vi "Execute_Single_Process.vi"(0 "Tab Control":T5, 1 "MaskParam 2":refnum<vi>, 5 "Parameter":variant, 7 "ImageIn":T3, 9 "ExtractImageControl":T3, 11 "error in (no error)":errorcluster, 12 "OperatorImage":T3) -> (3 "MaskParam 4":refnum<vi>, 4 "ProcessSettingOut":T6={"Enum_PreProcess"=enum."CamAttributes", "Parameter"=""}, 6 "ExtractImage":T3, 10 "Image Out":T3(plugin-control), 14 "OperatorImageOut":T3, 15 "error out":errorcluster)   [LabVIEW 2019]
uses:
  <vilib>/vision/NI_Vision_Development_Module.lvlib
  Controls/Process_Setting.ctl
  Controls/OperatorsParam_Type.ctl
  Controls/GrayMorphologyParam_Type.ctl
  Controls/LookupTableParam.ctl
  Controls/ParticleFilterParam_Type.ctl
  Controls/MaskParam_Type.ctl
  Ctrl/VisionProcessName.ctl
  <vilib>/vision/Image Controls.llb/IMAQ Image.ctl
  Controls/UI_Process_Type.ctl
  Controls/FiltersParam_Type.ctl
  Controls/BinaryMonoParam_Type.ctl
  Controls/ExtractPlanParam_Type.ctl
panel:
  in  "ExtractPlanParam":T1={"Color Plane"=enum."Green"}
  in  "BinaryMonoParam 2":T2={"Look For"=enum."Bright Objects", "Threshold"={136.0, 255.0}} {"Threshold" scale=0.0..255.0}
  in  "FiltersParam":T4={"Kernel"=[[1.0, 1.0, 1.0], [1.0, 1.0, 1.0], [1.0, 1.0, 1.0]], "Kernel Size"=0, "Filter Size X"=0, "Filter Size Y"=0, "Tolerance %"=0, "Divider"=0.0, "FilterFunction"=enum."Smoothing - Low Pass", "Sigma"=0.0, "LThres"=0.0, "HThresh"=0.0, "Windows Size"=0} {"Kernel Size" min=3 max=7 step=2}
  # "Minimum"
  # "Maximum"
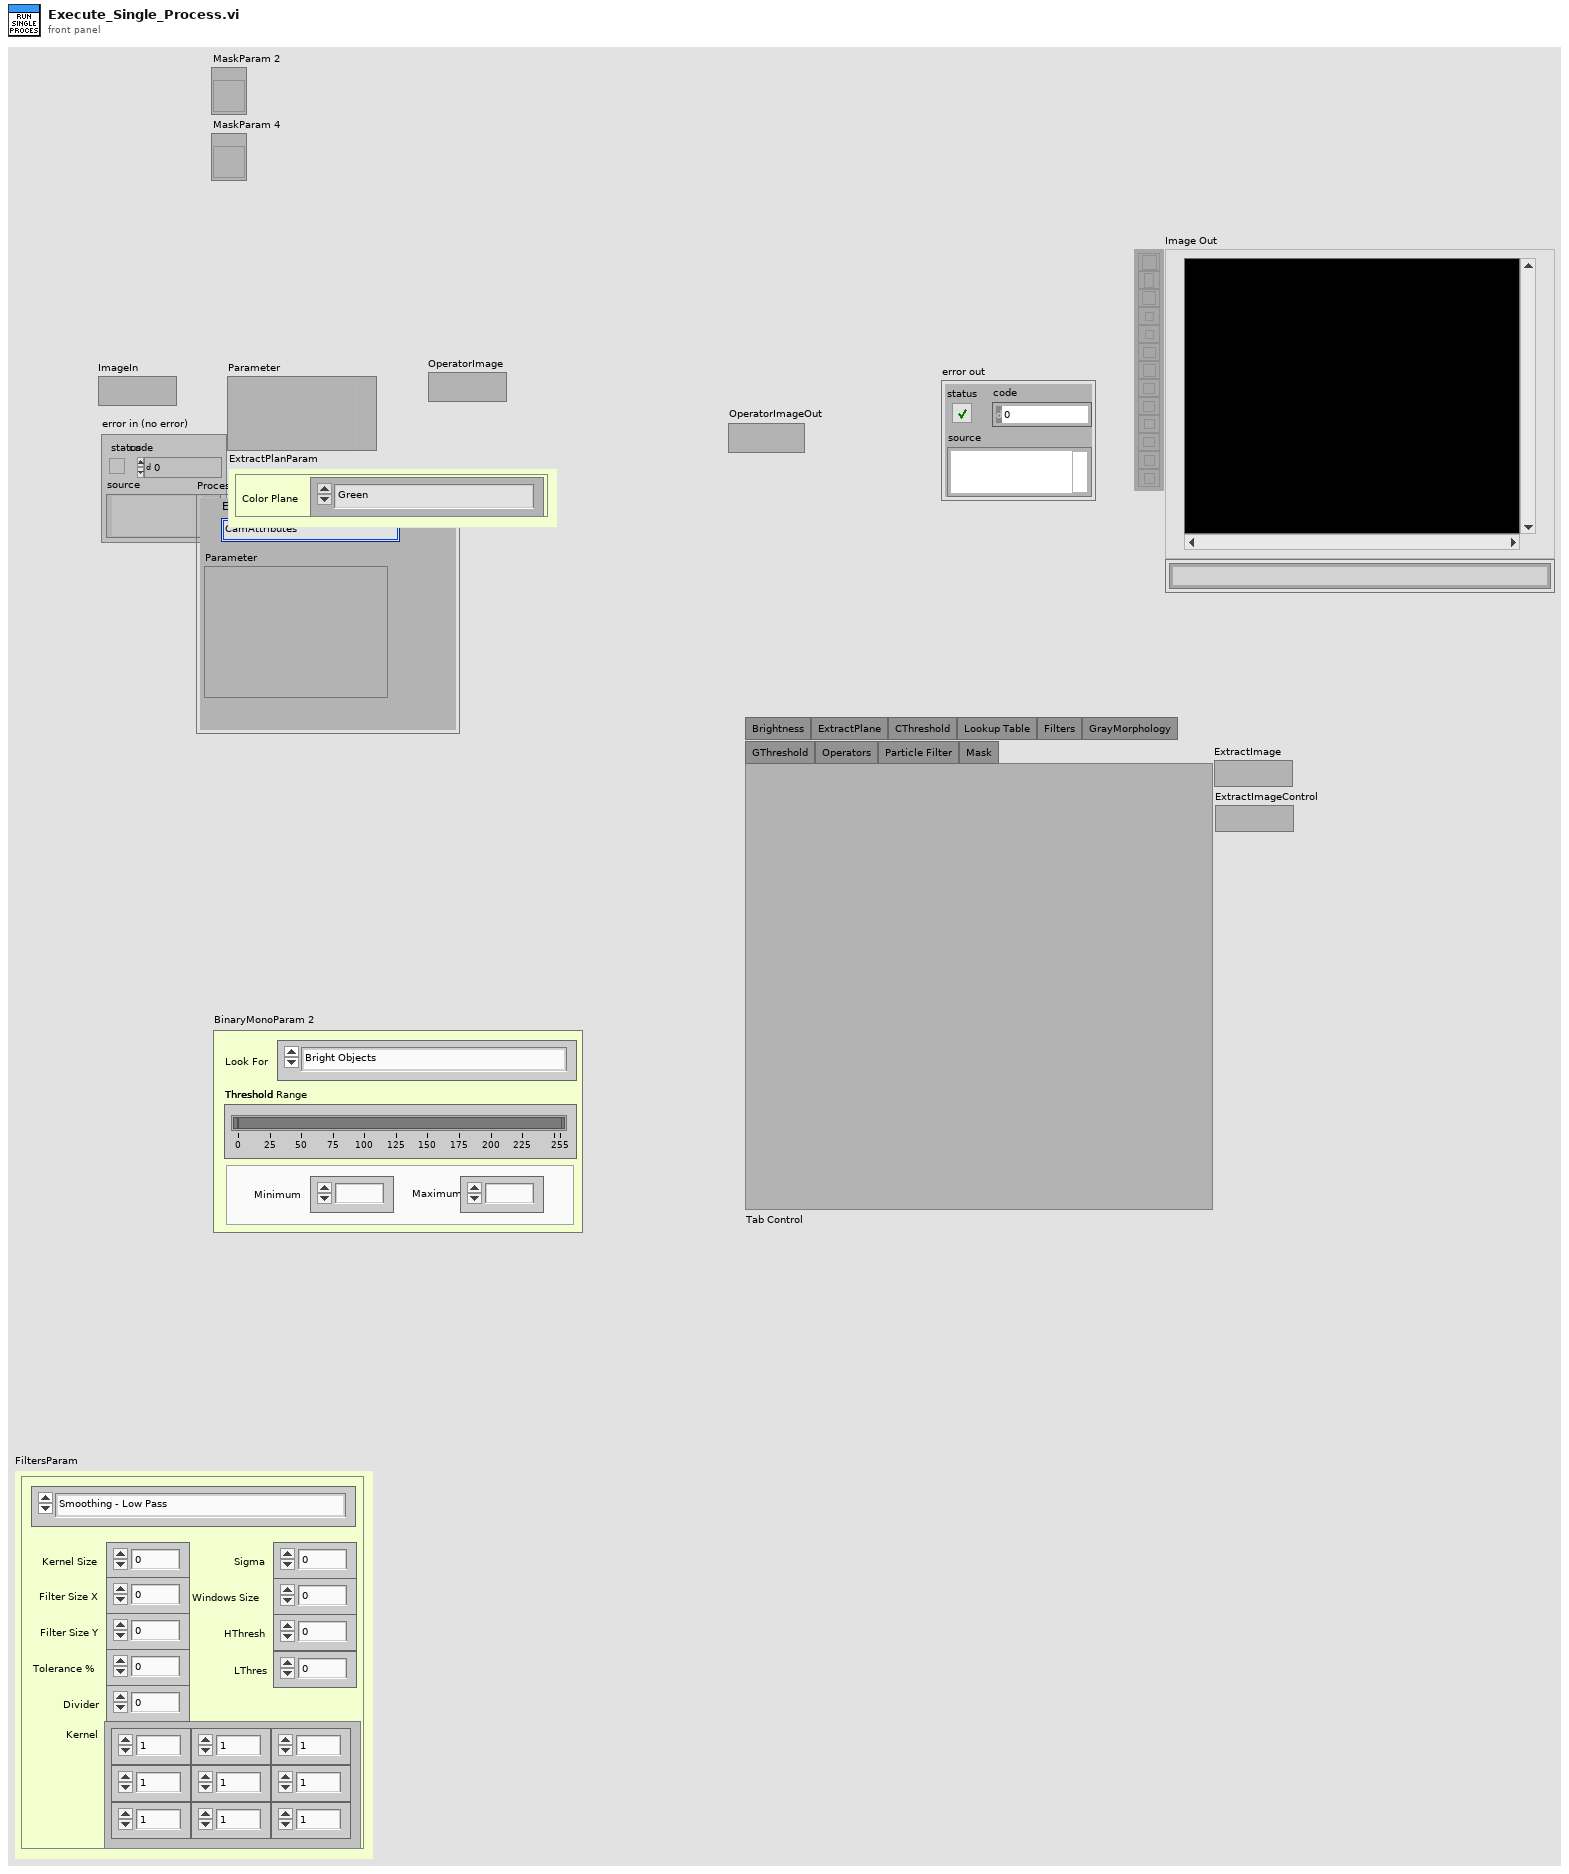
[diagram p1: front panel]
types:
  T1 = typedef "ExtractPlanParam_Type.ctl" = cluster{"Color Plane":enum16{"Red", "Green", "Blue", "Hue", "Saturation", "Luminance", "Value", "Intensity"}}
  T2 = typedef "BinaryMonoParam_Type.ctl" = cluster{"Look For":enum16{"Bright Objects", "Dark Objects", "Gray Objects"}, "Threshold":cluster{dbl, dbl}}
  T3 = typedef "IMAQ Image.ctl" = refnum<image>
  T4 = typedef "FiltersParam_Type.ctl" = cluster{"Kernel":sgl[][], "Kernel Size":i32, "Filter Size X":i32, "Filter Size Y":i32, "Tolerance %":i32, "Divider":sgl, "FilterFunction":enum16{"Smoothing - Low Pass", "Smoothing - Local Average", "Smoothing - Guassian", "Smoothing - Median", "------------------------------------", "Edge Detection - Laplacian", "Edge Detection - Diff", "Edge Detection - Prewitt", "Edge Detection - Sobel", "Edge Detection - Roberts", "Edge Detection - Canny", "Edge Detection - Gradient", "Edge Detection - Sigma", "----------------------------------------", "Convolution - Highlight Details", "Convolution - Custom"}, "Sigma":sgl, "LThres":sgl, "HThresh":sgl, "Windows Size":i32}
  T5 = typedef "UI_Process_Type.ctl" = enum32{"None", "Brightness", "ExtractPlane", "CThreshold", "Lookup Table", "Filters", "GrayMorphology", "GThreshold", "Operators", "Particle Filter", "Mask"}
  T6 = typedef "Process_Setting.ctl" = cluster{"Enum_PreProcess":T7, "Parameter":string}
  T7 = typedef "VisionProcessName.ctl" = enum16{"*CamParameter*", "CamAttributes", "*Preprocess*", "CG_Brightness", "C_Plane Extraction", "C_Threshold", "G_Lookup Table", "G_Threshold"}
  T8 = typedef "OperatorsParam_Type.ctl" = cluster{"Actions":enum16{"Add", "Subtract", "Multiply", "Divide", "Multiply Divide", "Modulo", "Absolutio Difference", "---------------------------------", "And", "Not And", "Or", "Not Or", "Exclusive Or", "Not Exclusive Or", "Logical Difference", "----------------------------------", "Mask"}, "Select Mode:":enum32{"Constant", "Image"}, "Color Box":u32, "Image Path":path}
  T9 = typedef "GrayMorphologyParam_Type.ctl" = cluster{"Operation":enum32{"AutoM", "Close", "Dilate", "Erode", "Gradient", "Gradient in", "Gradient out", "HitMiss", "Open", "PClose", "POpen", "Thick", "Thin"}, "Structuring Element":i32[][], "Square/Hexa (Square)":bool, "Number of iterations":i32}
  T10 = enum32{"Differentiation", "Gradient", "Prewitt", "Roberts", "Sigma", "Sobel"}
  T11 = typedef "LookupTableParam.ctl" = cluster{"Function":enum16{"Equalizer", "Reverse", "Logarithmic", "Exponential", "Square", "Square Root", "Power X", "Power 1/X"}, "Power Value":sgl}
  T12 = enum32{"Linear", "Log", "Exp", "Square", "Square root", "Power X", "Power 1/X"}
  T13 = typedef "ParticleFilterParam_Type.ctl" = cluster{"Selection Values":cluster{"Measurement Parameter":T14, "Range Lower Value":dbl, "Range Upper Value":dbl, "Range":bool, "Measurement Type":bool}[], "Keep/Remove Particles (F)":bool, "Reject Border? (F)":bool, "Fill Holes? (F)":bool, "Connectivity 4/8 (8)":bool}
  T14 = typedef "Particle Parameters" = i32
  T15 = enum16{"Red", "Green", "Blue", "Hue", "Saturation", "Luminance", "Value", "Intensity"}
  T16 = enum16{"Add", "Subtract", "Multiply", "Divide", "Multiply Divide", "Modulo", "Absolutio Difference", "---------------------------------", "And", "Not And", "Or", "Not Or", "Exclusive Or", "Not Exclusive Or", "Logical Difference", "----------------------------------", "Mask"}
  T17 = enum32{"AutoM", "Close", "Dilate", "Erode", "Gradient", "Gradient in", "Gradient out", "HitMiss", "Open", "PClose", "POpen", "Thick", "Thin"}
  T18 = enum16{"Smoothing - Low Pass", "Smoothing - Local Average", "Smoothing - Guassian", "Smoothing - Median", "------------------------------------", "Edge Detection - Laplacian", "Edge Detection - Diff", "Edge Detection - Prewitt", "Edge Detection - Sobel", "Edge Detection - Roberts", "Edge Detection - Canny", "Edge Detection - Gradient", "Edge Detection - Sigma", "----------------------------------------", "Convolution - Highlight Details", "Convolution - Custom"}
  T19 = cluster{"Filter Size X":i32, "Filter Size Y":i32, "Tolerance %":i32}
  T20 = cluster{"Filter Size X":i32, "Filter Size Y":i32, dbl}
  T21 = cluster{"Sigma":sgl, "HThresh":sgl, "LThres":sgl, "WindowSize":i32}
  T22 = enum16{"Equalizer", "Reverse", "Logarithmic", "Exponential", "Square", "Square Root", "Power X", "Power 1/X"}
  T23 = cluster{"histogram":u32[], "Minimal Value":sgl, "Maximal Value":sgl, "Starting Value":sgl, "Interval Width":sgl, "Mean Value":sgl, "Standard  Variation":sgl, "Area (pixels)":i32}
  T24 = typedef "Image Type" = u32
  T25 = cluster{"Measurement Parameter":T14, "Range Lower Value":dbl, "Range Upper Value":dbl, "Range":bool, "Measurement Type":bool}[]
  T26 = typedef "MaskParam_Type.ctl" = cluster{"Function":enum16{"Inside", "Outside"}, "ROI List":i32, "ROI":cluster{"Global Rectangle":i32[], "Contours":cluster{"Contour Type":u32, "ROI Type":u32, "Points":i32[]}[]}[], "Creat ROI":bool, "Delete ROI":bool, "Enabled/Disabled":bool, "Color Box":u32, "Last Mouse Position":cluster{"X":i32, "Y":i32}}
  T27 = cluster{"Global Rectangle":i32[], "Contours":cluster{"Contour Type":u32, "ROI Type":u32, "Points":i32[]}[]}[]
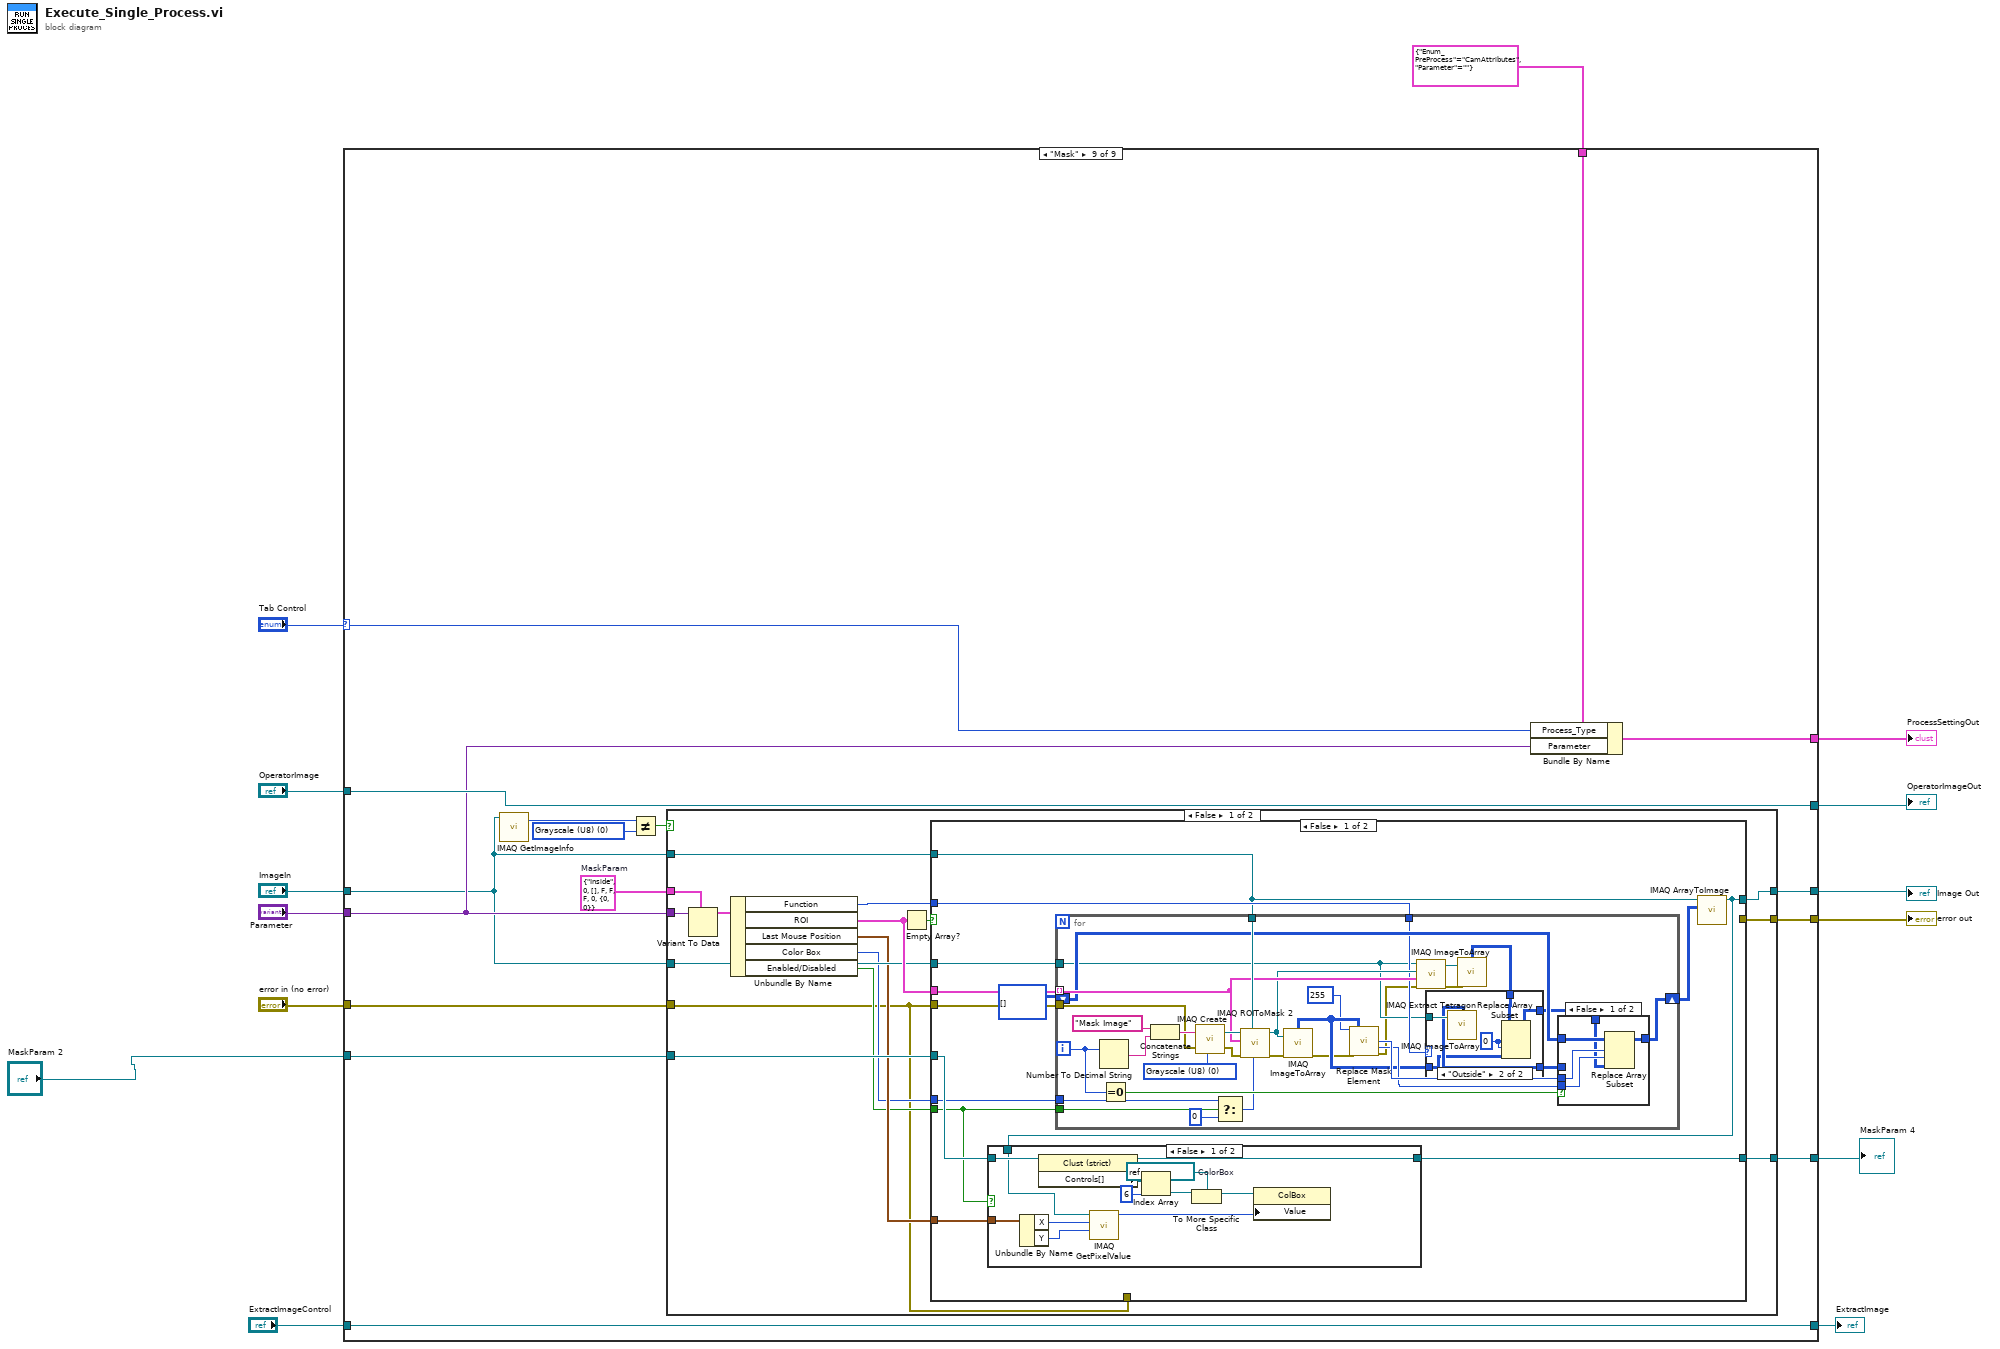
[diagram p0: block diagram]
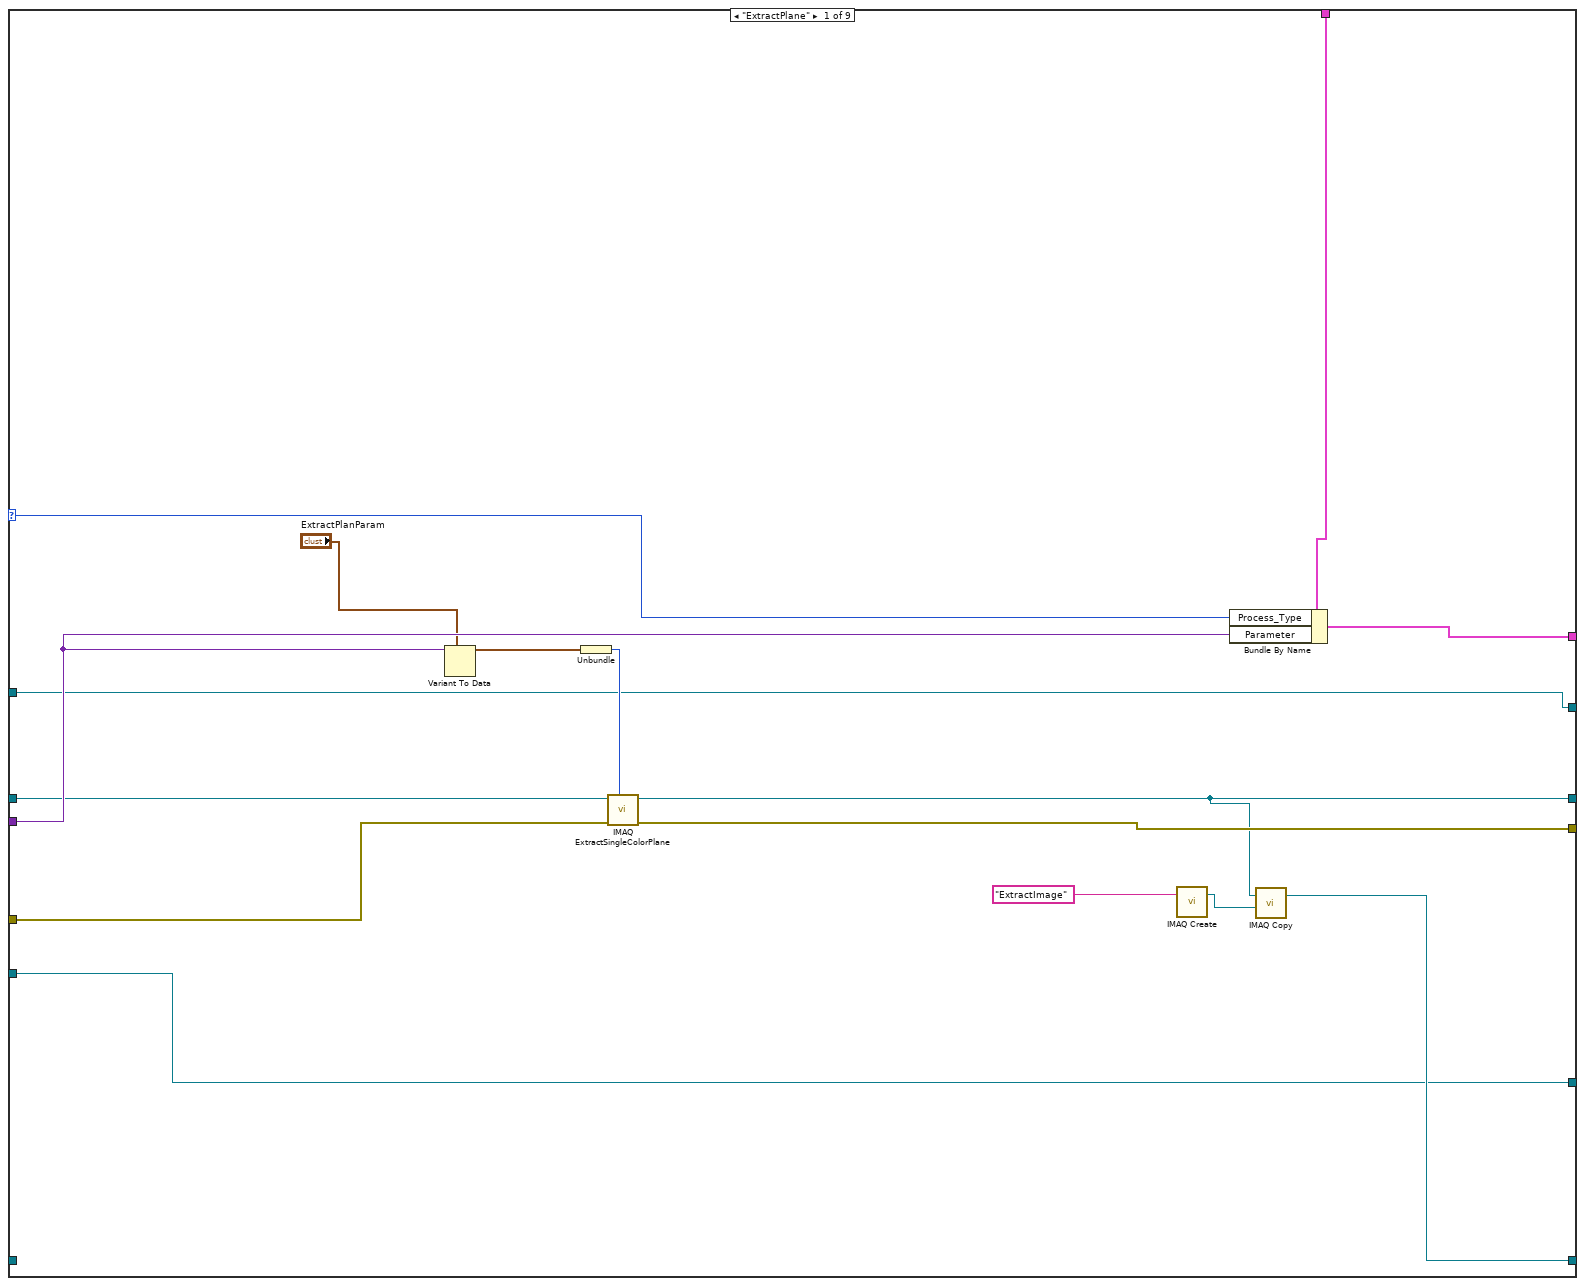
[diagram p2: hidden frame]
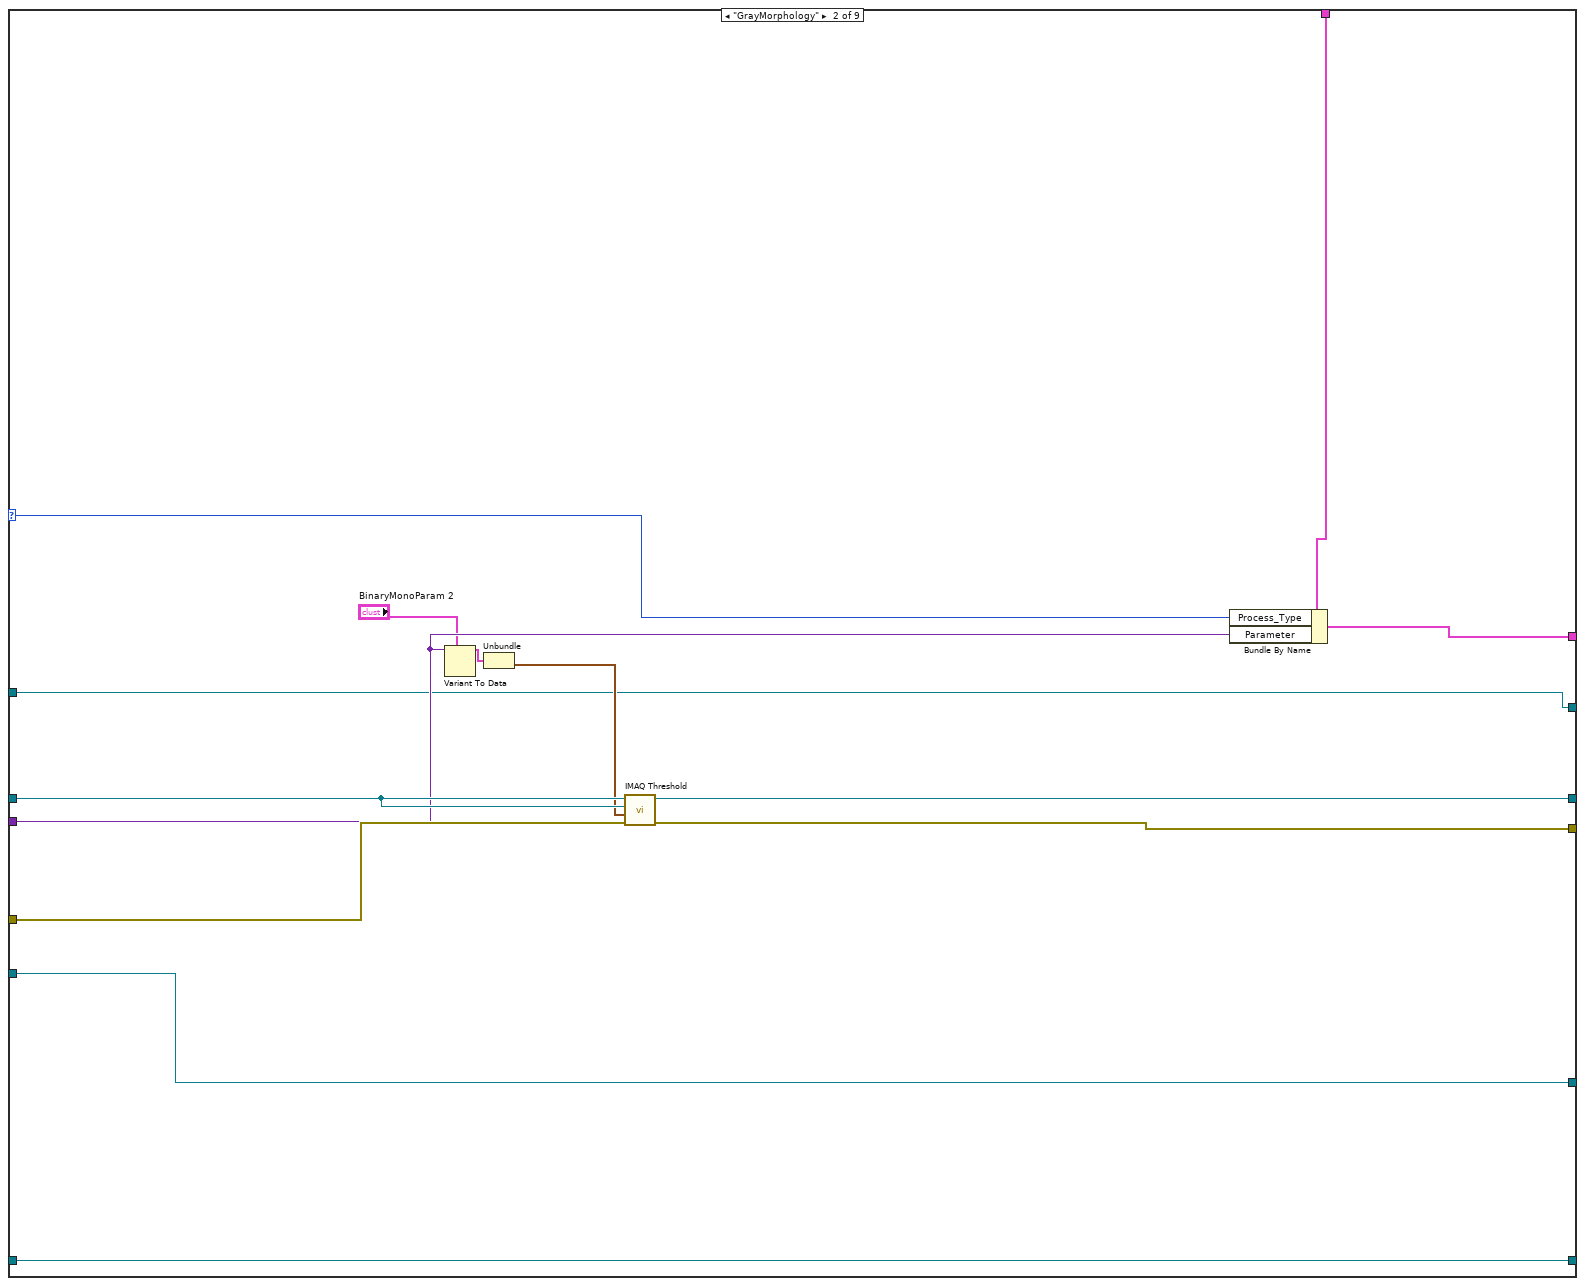
[diagram p3: hidden frame]
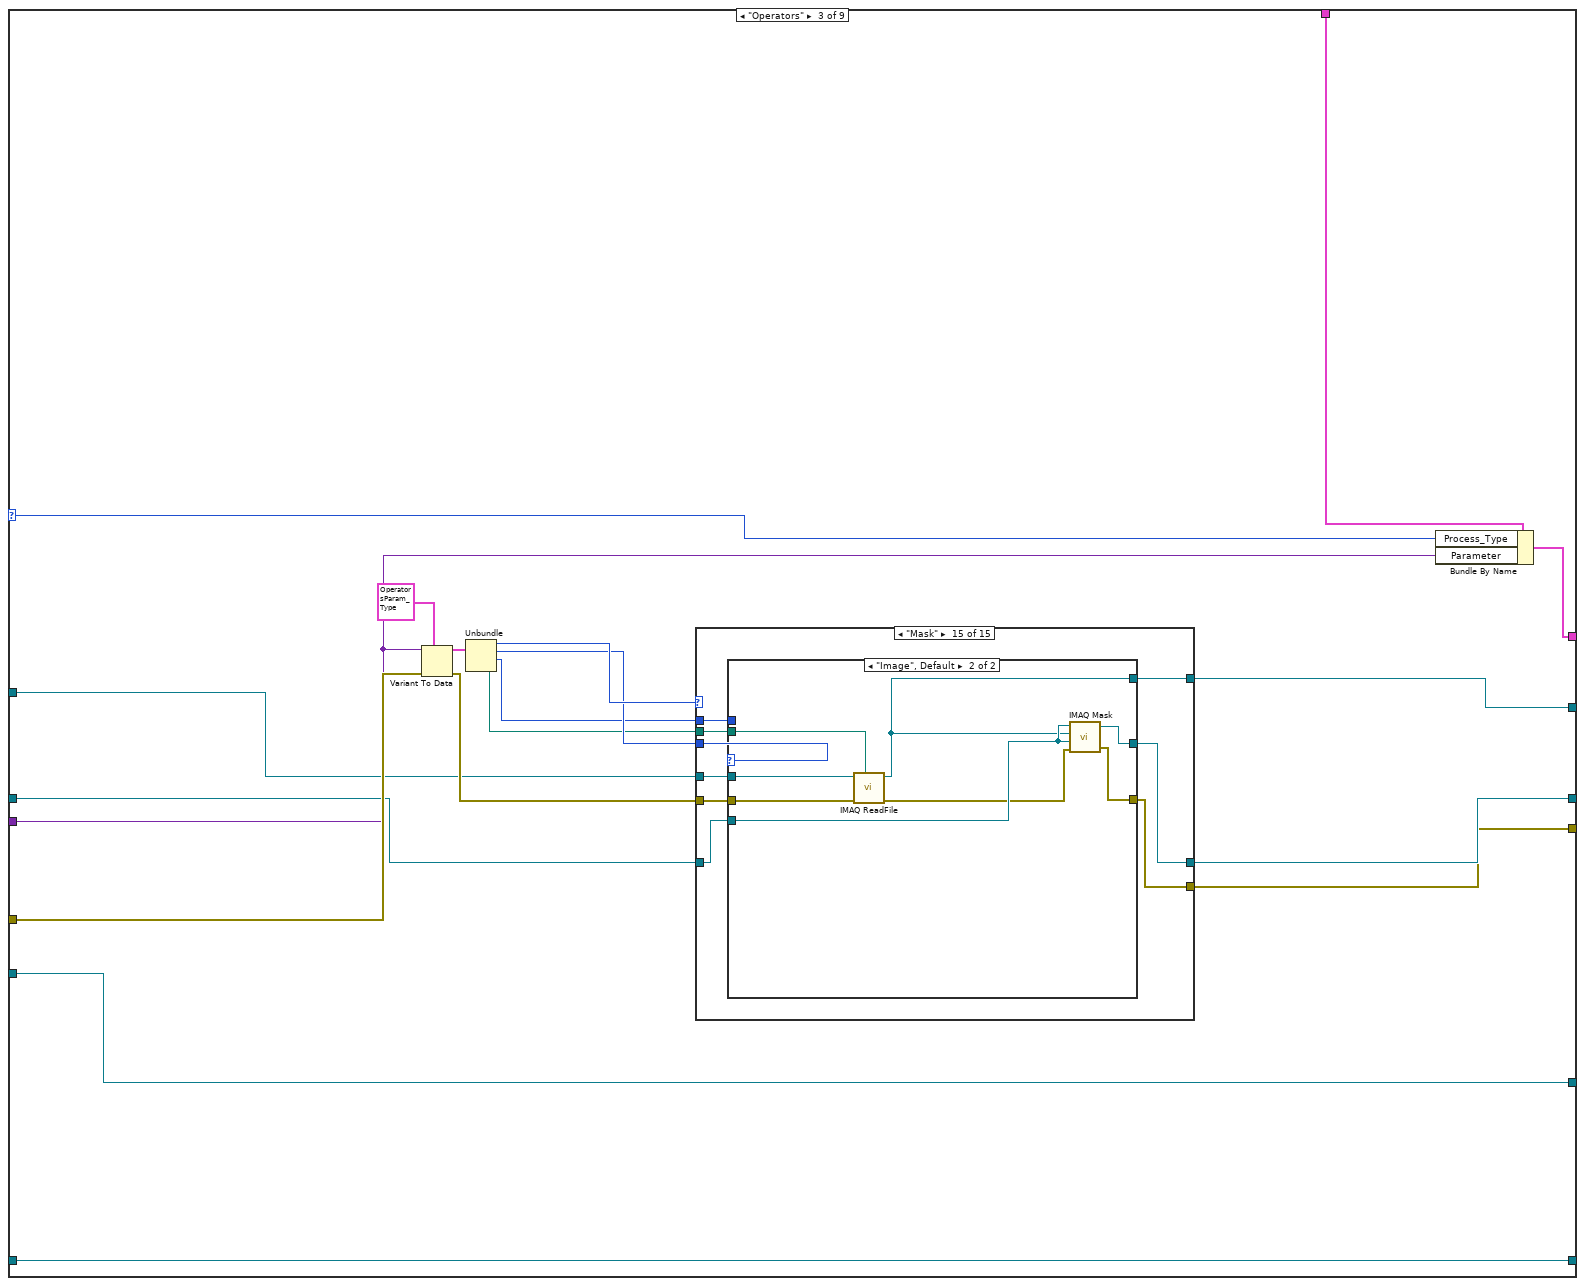
[diagram p4: hidden frame]
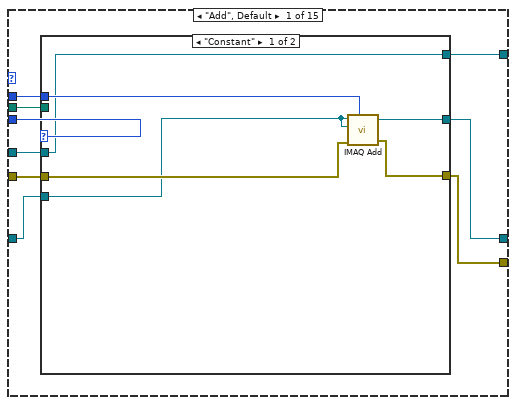
[diagram p5: hidden frame]
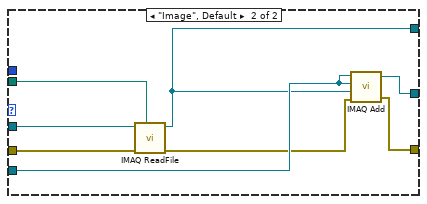
[diagram p6: hidden frame]
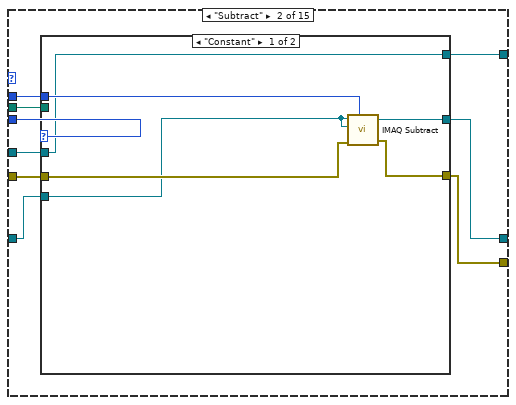
[diagram p7: hidden frame]
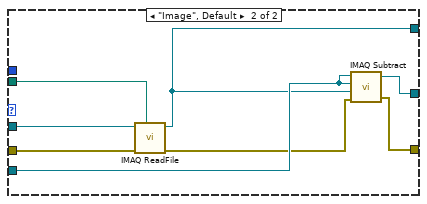
[diagram p8: hidden frame]
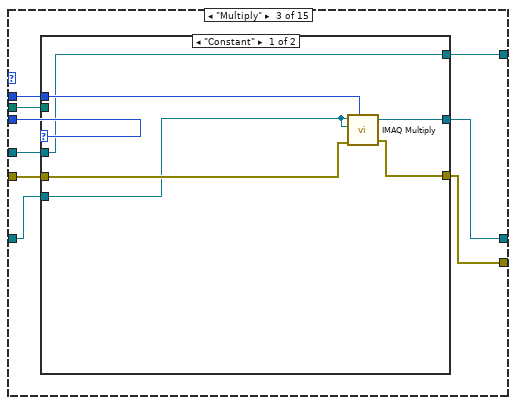
[diagram p9: hidden frame]
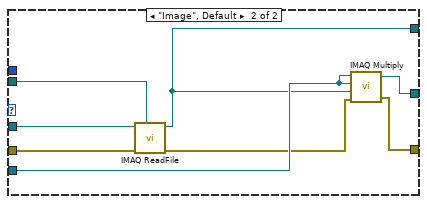
[diagram p10: hidden frame]
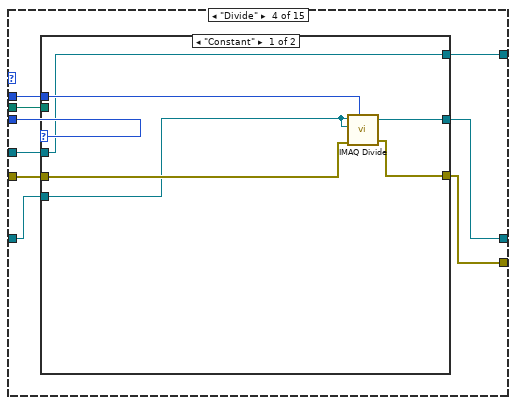
[diagram p11: hidden frame]
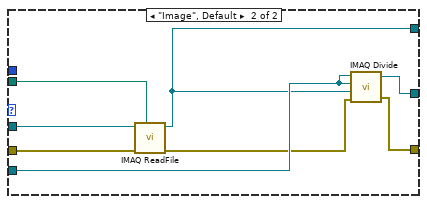
[diagram p12: hidden frame]
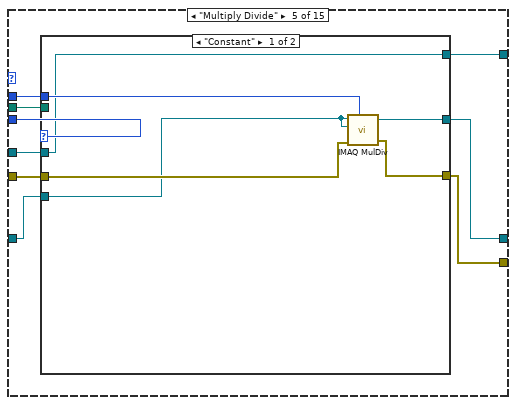
[diagram p13: hidden frame]
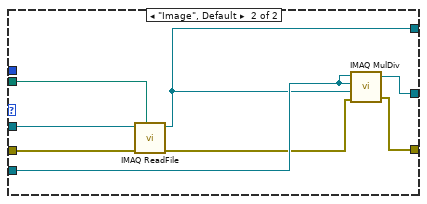
[diagram p14: hidden frame]
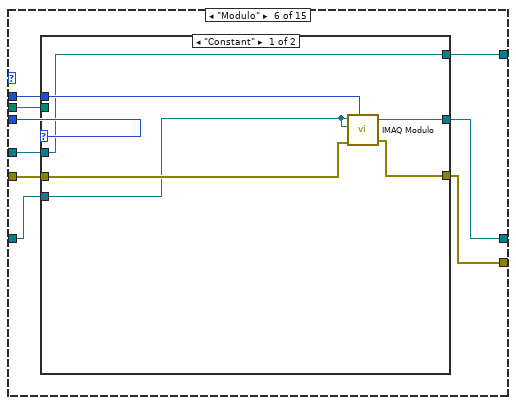
[diagram p15: hidden frame]
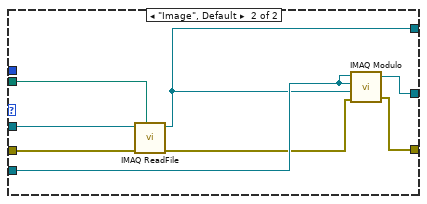
[diagram p16: hidden frame]
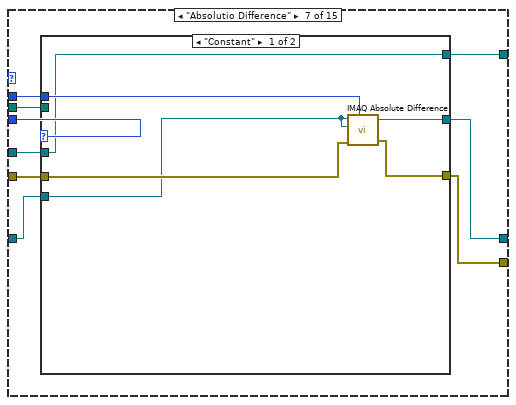
[diagram p17: hidden frame]
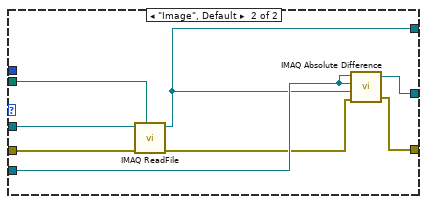
[diagram p18: hidden frame]
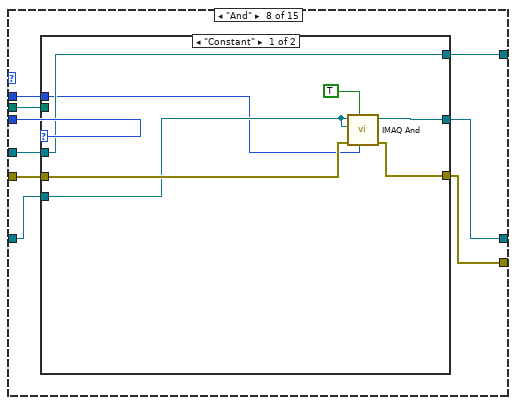
[diagram p19: hidden frame]
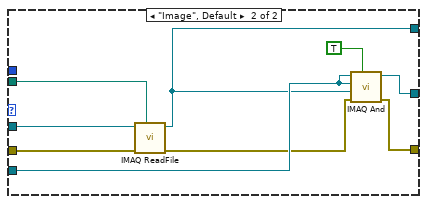
[diagram p20: hidden frame]
diagram:
  n1 = case shown="\"Mask\"" "Tab Control" {
    selector: "Tab Control" -> [w26 w42 w51 w423 w456 w584 w661 _ w680]
    tunnel: "ImageIn" -> [w22 w39 w60 w426 w448 w592 w657 w672 w673]
    tunnel: [w18 w38 w57 w425 w447 w589 w658 w672 w687] -> w10
    tunnel: T6 {"Enum_PreProcess"=enum."CamAttributes", "Parameter"=""} ("ProcessSetting") -> [w30 w44 w52 w424 w457 w587 w664 _ w682]
    tunnel: [w29 w43 w49 w422 w455 w586 w663 _ w681] -> w9
    tunnel: [w28 w40 w54 w427 w449 w590 w654 w671 w685] -> w11
    tunnel: "error in (no error)" -> [w27 w41 w63 w428 w450 w596 w666 w671 w686]
    tunnel: "Parameter" -> [w23 w35 w50 w420 w435 w585 w662 _ w679]
    tunnel: "OperatorImage" -> [w21 w34 w48 w434 w458 w597 w667 w670 w688]
    tunnel: [w21 w34 w47 w434 w458 w597 w667 w670 w688] -> w5
    tunnel: [w17 w33 w46 w419 w439 w583 w650 w669 w677] -> w4
    tunnel: "ExtractImageControl" -> [_ w33 w46 w419 w439 w583 w650 w669 w677]
    tunnel: "MaskParam 2" -> [w16 w32 w45 w418 w438 w582 w649 w668 w675]
    tunnel: [w16 w32 w45 w418 w438 w582 w649 w668 w674] -> w1
    frame "ExtractPlane" {
      n2 = Variant To Data(type="ExtractPlanParam", Variant=w23) -> (data=w25:T1)  [unwired: 1 in, 1 out]
      n3 = Unbundle(w25) -> ("Color Plane"=w24:T15)
      n4 = call "IMAQ ExtractSingleColorPlane"("Color Plane"=w24, "error in (no error)"=w27, "Image Src"=w22) -> ("error out"=w28:errorcluster, "Image Dst Out"=w18:T3)  [unwired: 7 in]
      n5 = call "IMAQ Create"("Image Name"="ExtractImage") -> ("New Image"=w19:T3)  [unwired: 4 in, 1 out]
      n6 = Bundle By Name(cluster=w30, "Process_Type"=w26, "Parameter"=w23) -> (w29:T6)
      n7 = call "IMAQ Copy"("Image Dst"=w19, "Image Src"=w18) -> ("Image Dst Out"=w17:T3)  [unwired: 4 in, 1 out]
    }
    frame "GrayMorphology" {
      n8 = Variant To Data(type="BinaryMonoParam 2", Variant=w35) -> (data=w37:T2)  [unwired: 1 in, 1 out]
      n9 = Unbundle(w37) -> ("Threshold"=w36:cluster{dbl, dbl})  [unwired: 1 out]
      n10 = call "IMAQ Threshold"("error in (no error)"=w41, "Range"=w36, "Image Dst"=w39, "Image Src"=w39) -> ("error out"=w40:errorcluster, "Image Dst Out"=w38:T3)  [unwired: 2 in, 4 out]
      n11 = Bundle By Name(cluster=w44, "Process_Type"=w42, "Parameter"=w35) -> (w43:T6)
    }
    frame "Operators" {
      n12 = Variant To Data(error in=w63, type=T8 {"Actions"=enum."Add", "Select Mode:"=enum."Image", "Color Box"=0, "Image Path"=path "\\\\Mac\\Home/Desktop/ssss.png"} ("OperatorsParam"), Variant=w50) -> (data=w62:T8, error out=w55:errorcluster)
      n13 = Unbundle(w62) -> ("Actions"=w61:T16, "Select Mode:"=w59:enum32{"Constant", "Image"}, "Color Box"=w58:u32, "Image Path"=w56:path)
      n14 = case shown="\"Mask\"" w61 {
        tunnel: w60 -> [w71 w94 w117 w140 w163 w186 w209 w232 w257 w282 w307 w332 w357 w382 w405]
        tunnel: w59 -> [w68 w91 w114 w137 w160 w183 w206 w229 w254 w279 w304 w329 w354 w379 w402]
        tunnel: w58 -> [w72 w95 w118 w141 w164 w187 w210 w233 w258 w283 w308 w333 w358 w383 w406]
        tunnel: [w70 w93 w116 w139 w162 w185 w208 w231 w256 w281 w306 w331 w356 w381 w404] -> w57
        tunnel: w56 -> [w69 w92 w115 w138 w161 w184 w207 w230 w255 w280 w305 w330 w355 w380 w403]
        tunnel: w55 -> [w67 w90 w113 w136 w159 w182 w205 w228 w253 w278 w303 w328 w353 w378 w401]
        tunnel: [w66 w89 w112 w135 w158 w181 w204 w227 w252 w277 w302 w327 w352 w377 w400] -> w54
        tunnel: [w65 w88 w111 w134 w157 w180 w203 w226 w251 w276 w301 w326 w351 w376 w399] -> w47
        tunnel: w48 -> [w64 w87 w110 w133 w156 w179 w202 w225 w250 w275 w300 w325 w350 w375 w398]
        frame "Add", Default {
          n15 = case shown="\"Constant\"" w68 {
            tunnel: w72 -> [w78 _]
            tunnel: w71 -> [w74 w86]
            tunnel: [w75 w85] -> w70
            tunnel: w69 -> [_ w84]
            tunnel: w67 -> [w77 w81]
            tunnel: [w76 w82] -> w66
            tunnel: [w73 w80] -> w65
            tunnel: w64 -> [w73 w79]
            frame "Constant" {
              n16 = call "IMAQ Add"("Image Src A"=w74, "Constant"=w78, "Image Dst"=w74, "error in (no error)"=w77) -> ("Image Dst Out"=w75:T3, "error out"=w76:errorcluster)  [unwired: 3 in]
            }
            frame "Image", Default {
              n17 = call "IMAQ ReadFile"("File Path"=w84, "error in (no error)"=w81, "Image"=w79) -> ("error out"=w83:errorcluster, "Image Out"=w80:T3)  [unwired: 4 in, 3 out]
              n18 = call "IMAQ Add"("Image Src A"=w86, "Image Dst"=w86, "Image Src B"=w80, "error in (no error)"=w83) -> ("Image Dst Out"=w85:T3, "error out"=w82:errorcluster)  [unwired: 3 in]
            }
          }
        }
        frame "Subtract" {
          n19 = case shown="\"Constant\"" w91 {
            tunnel: w95 -> [w101 _]
            tunnel: w94 -> [w97 w109]
            tunnel: [w98 w108] -> w93
            tunnel: w92 -> [_ w107]
            tunnel: w90 -> [w100 w104]
            tunnel: [w99 w105] -> w89
            tunnel: [w96 w103] -> w88
            tunnel: w87 -> [w96 w102]
            frame "Constant" {
              n20 = call "IMAQ Subtract"("Image Src A"=w97, "Constant"=w101, "Image Dst"=w97, "error in (no error)"=w100) -> ("Image Dst Out"=w98:T3, "error out"=w99:errorcluster)  [unwired: 3 in]
            }
            frame "Image", Default {
              n21 = call "IMAQ ReadFile"("File Path"=w107, "error in (no error)"=w104, "Image"=w102) -> ("error out"=w106:errorcluster, "Image Out"=w103:T3)  [unwired: 4 in, 3 out]
              n22 = call "IMAQ Subtract"("Image Src A"=w109, "Image Dst"=w109, "Image Src B"=w103, "error in (no error)"=w106) -> ("Image Dst Out"=w108:T3, "error out"=w105:errorcluster)  [unwired: 3 in]
            }
          }
        }
        frame "Multiply" {
          n23 = case shown="\"Constant\"" w114 {
            tunnel: w118 -> [w124 _]
            tunnel: w117 -> [w120 w132]
            tunnel: [w121 w131] -> w116
            tunnel: w115 -> [_ w130]
            tunnel: w113 -> [w123 w127]
            tunnel: [w122 w128] -> w112
            tunnel: [w119 w126] -> w111
            tunnel: w110 -> [w119 w125]
            frame "Constant" {
              n24 = call "IMAQ Multiply"("Image Src A"=w120, "Constant"=w124, "Image Dst"=w120, "error in (no error)"=w123) -> ("Image Dst Out"=w121:T3, "error out"=w122:errorcluster)  [unwired: 3 in]
            }
            frame "Image", Default {
              n25 = call "IMAQ ReadFile"("File Path"=w130, "error in (no error)"=w127, "Image"=w125) -> ("error out"=w129:errorcluster, "Image Out"=w126:T3)  [unwired: 4 in, 3 out]
              n26 = call "IMAQ Multiply"("Image Src A"=w132, "Image Dst"=w132, "Image Src B"=w126, "error in (no error)"=w129) -> ("Image Dst Out"=w131:T3, "error out"=w128:errorcluster)  [unwired: 3 in]
            }
          }
        }
        frame "Divide" {
          n27 = case shown="\"Constant\"" w137 {
            tunnel: w141 -> [w147 _]
            tunnel: w140 -> [w143 w155]
            tunnel: [w144 w154] -> w139
            tunnel: w138 -> [_ w153]
            tunnel: w136 -> [w146 w150]
            tunnel: [w145 w151] -> w135
            tunnel: [w142 w149] -> w134
            tunnel: w133 -> [w142 w148]
            frame "Constant" {
              n28 = call "IMAQ Divide"("Image Src A"=w143, "Constant"=w147, "Image Dst"=w143, "error in (no error)"=w146) -> ("Image Dst Out"=w144:T3, "error out"=w145:errorcluster)  [unwired: 3 in]
            }
            frame "Image", Default {
              n29 = call "IMAQ ReadFile"("File Path"=w153, "error in (no error)"=w150, "Image"=w148) -> ("error out"=w152:errorcluster, "Image Out"=w149:T3)  [unwired: 4 in, 3 out]
              n30 = call "IMAQ Divide"("Image Src A"=w155, "Image Dst"=w155, "Image Src B"=w149, "error in (no error)"=w152) -> ("Image Dst Out"=w154:T3, "error out"=w151:errorcluster)  [unwired: 3 in]
            }
          }
        }
        frame "Multiply Divide" {
          n31 = case shown="\"Constant\"" w160 {
            tunnel: w164 -> [w170 _]
            tunnel: w163 -> [w166 w178]
            tunnel: [w167 w177] -> w162
            tunnel: w161 -> [_ w176]
            tunnel: w159 -> [w169 w173]
            tunnel: [w168 w174] -> w158
            tunnel: [w165 w172] -> w157
            tunnel: w156 -> [w165 w171]
            frame "Constant" {
              n32 = call "IMAQ MulDiv"("Image Src A"=w166, "Constant"=w170, "Image Dst"=w166, "error in (no error)"=w169) -> ("Image Dst Out"=w167:T3, "error out"=w168:errorcluster)  [unwired: 3 in]
            }
            frame "Image", Default {
              n33 = call "IMAQ ReadFile"("File Path"=w176, "error in (no error)"=w173, "Image"=w171) -> ("error out"=w175:errorcluster, "Image Out"=w172:T3)  [unwired: 4 in, 3 out]
              n34 = call "IMAQ MulDiv"("Image Src A"=w178, "Image Dst"=w178, "Image Src B"=w172, "error in (no error)"=w175) -> ("Image Dst Out"=w177:T3, "error out"=w174:errorcluster)  [unwired: 3 in]
            }
          }
        }
        frame "Modulo" {
          n35 = case shown="\"Constant\"" w183 {
            tunnel: w187 -> [w193 _]
            tunnel: w186 -> [w189 w201]
            tunnel: [w190 w200] -> w185
            tunnel: w184 -> [_ w199]
            tunnel: w182 -> [w192 w196]
            tunnel: [w191 w197] -> w181
            tunnel: [w188 w195] -> w180
            tunnel: w179 -> [w188 w194]
            frame "Constant" {
              n36 = call "IMAQ Modulo"("Image Src A"=w189, "Constant"=w193, "Image Dst"=w189, "error in (no error)"=w192) -> ("Image Dst Out"=w190:T3, "error out"=w191:errorcluster)  [unwired: 3 in]
            }
            frame "Image", Default {
              n37 = call "IMAQ ReadFile"("File Path"=w199, "error in (no error)"=w196, "Image"=w194) -> ("error out"=w198:errorcluster, "Image Out"=w195:T3)  [unwired: 4 in, 3 out]
              n38 = call "IMAQ Modulo"("Image Src A"=w201, "Image Dst"=w201, "Image Src B"=w195, "error in (no error)"=w198) -> ("Image Dst Out"=w200:T3, "error out"=w197:errorcluster)  [unwired: 3 in]
            }
          }
        }
        frame "Absolutio Difference" {
          n39 = case shown="\"Constant\"" w206 {
            tunnel: w210 -> [w216 _]
            tunnel: w209 -> [w212 w224]
            tunnel: [w213 w223] -> w208
            tunnel: w207 -> [_ w222]
            tunnel: w205 -> [w215 w219]
            tunnel: [w214 w220] -> w204
            tunnel: [w211 w218] -> w203
            tunnel: w202 -> [w211 w217]
            frame "Constant" {
              n40 = call "IMAQ Absolute Difference"("Image Src A"=w212, "Constant"=w216, "Image Dst"=w212, "error in (no error)"=w215) -> ("Image Dst Out"=w213:T3, "error out"=w214:errorcluster)  [unwired: 3 in]
            }
            frame "Image", Default {
              n41 = call "IMAQ ReadFile"("File Path"=w222, "error in (no error)"=w219, "Image"=w217) -> ("error out"=w221:errorcluster, "Image Out"=w218:T3)  [unwired: 4 in, 3 out]
              n42 = call "IMAQ Absolute Difference"("Image Src A"=w224, "Image Dst"=w224, "Image Src B"=w218, "error in (no error)"=w221) -> ("Image Dst Out"=w223:T3, "error out"=w220:errorcluster)  [unwired: 3 in]
            }
          }
        }
        frame "And" {
          n43 = case shown="\"Constant\"" w229 {
            tunnel: w233 -> [w235 _]
            tunnel: w232 -> [w237 w249]
            tunnel: [w238 w248] -> w231
            tunnel: w230 -> [_ w247]
            tunnel: w228 -> [w240 w244]
            tunnel: [w239 w245] -> w227
            tunnel: [w236 w243] -> w226
            tunnel: w225 -> [w236 w242]
            frame "Constant" {
              n44 = call "IMAQ And"("Constant"=w235, "And/Nand (And)"=TRUE, "error in (no error)"=w240, "Image Dst"=w237, "Image Src A"=w237) -> ("error out"=w239:errorcluster, "Image Dst Out"=w238:T3)  [unwired: 5 in]
            }
            frame "Image", Default {
              n45 = call "IMAQ ReadFile"("File Path"=w247, "error in (no error)"=w244, "Image"=w242) -> ("error out"=w246:errorcluster, "Image Out"=w243:T3)  [unwired: 4 in, 3 out]
              n46 = call "IMAQ And"("And/Nand (And)"=TRUE, "error in (no error)"=w246, "Image Src B"=w243, "Image Dst"=w249, "Image Src A"=w249) -> ("error out"=w245:errorcluster, "Image Dst Out"=w248:T3)  [unwired: 5 in]
            }
          }
        }
        frame "Not And" {
          n47 = case shown="\"Image\", Default" w254 {
            tunnel: w258 -> [w260 _]
            tunnel: w257 -> [w262 w274]
            tunnel: [w263 w273] -> w256
            tunnel: w255 -> [_ w272]
            tunnel: w253 -> [w265 w269]
            tunnel: [w264 w270] -> w252
            tunnel: [w261 w268] -> w251
            tunnel: w250 -> [w261 w267]
            frame "Constant" {
              n48 = call "IMAQ And"("Constant"=w260, "And/Nand (And)"=FALSE, "error in (no error)"=w265, "Image Dst"=w262, "Image Src A"=w262) -> ("error out"=w264:errorcluster, "Image Dst Out"=w263:T3)  [unwired: 5 in]
            }
            frame "Image", Default {
              n49 = call "IMAQ ReadFile"("File Path"=w272, "error in (no error)"=w269, "Image"=w267) -> ("error out"=w271:errorcluster, "Image Out"=w268:T3)  [unwired: 4 in, 3 out]
              n50 = call "IMAQ And"("And/Nand (And)"=FALSE, "error in (no error)"=w271, "Image Src B"=w268, "Image Dst"=w274, "Image Src A"=w274) -> ("error out"=w270:errorcluster, "Image Dst Out"=w273:T3)  [unwired: 5 in]
            }
          }
        }
        frame "Or" {
          n51 = case shown="\"Image\", Default" w279 {
            tunnel: w283 -> [w285 _]
            tunnel: w282 -> [w287 w299]
            tunnel: [w288 w298] -> w281
            tunnel: w280 -> [_ w297]
            tunnel: w278 -> [w290 w294]
            tunnel: [w289 w295] -> w277
            tunnel: [w286 w293] -> w276
            tunnel: w275 -> [w286 w292]
            frame "Constant" {
              n52 = call "IMAQ Or"("Constant"=w285, "Or/Nor (Or)"=TRUE ("And/Nand (And)"), "error in (no error)"=w290, "Image Dst"=w287, "Image Src A"=w287) -> ("error out"=w289:errorcluster, "Image Dst Out"=w288:T3)  [unwired: 5 in]
            }
            frame "Image", Default {
              n53 = call "IMAQ ReadFile"("File Path"=w297, "error in (no error)"=w294, "Image"=w292) -> ("error out"=w296:errorcluster, "Image Out"=w293:T3)  [unwired: 4 in, 3 out]
              n54 = call "IMAQ Or"("Or/Nor (Or)"=TRUE ("And/Nand (And)"), "error in (no error)"=w296, "Image Src B"=w293, "Image Dst"=w299, "Image Src A"=w299) -> ("error out"=w295:errorcluster, "Image Dst Out"=w298:T3)  [unwired: 5 in]
            }
          }
        }
        frame "Not Or" {
          n55 = case shown="\"Constant\"" w304 {
            tunnel: w308 -> [w310 _]
            tunnel: w307 -> [w312 w324]
            tunnel: [w313 w323] -> w306
            tunnel: w305 -> [_ w322]
            tunnel: w303 -> [w315 w319]
            tunnel: [w314 w320] -> w302
            tunnel: [w311 w318] -> w301
            tunnel: w300 -> [w311 w317]
            frame "Constant" {
              n56 = call "IMAQ Or"("Constant"=w310, "Or/Nor (Or)"=FALSE ("And/Nand (And)"), "error in (no error)"=w315, "Image Dst"=w312, "Image Src A"=w312) -> ("error out"=w314:errorcluster, "Image Dst Out"=w313:T3)  [unwired: 5 in]
            }
            frame "Image", Default {
              n57 = call "IMAQ ReadFile"("File Path"=w322, "error in (no error)"=w319, "Image"=w317) -> ("error out"=w321:errorcluster, "Image Out"=w318:T3)  [unwired: 4 in, 3 out]
              n58 = call "IMAQ Or"("Or/Nor (Or)"=FALSE ("And/Nand (And)"), "error in (no error)"=w321, "Image Src B"=w318, "Image Dst"=w324, "Image Src A"=w324) -> ("error out"=w320:errorcluster, "Image Dst Out"=w323:T3)  [unwired: 5 in]
            }
          }
        }
        frame "Exclusive Or" {
          n59 = case shown="\"Image\", Default" w329 {
            tunnel: w333 -> [w335 _]
            tunnel: w332 -> [w337 w349]
            tunnel: [w338 w348] -> w331
            tunnel: w330 -> [_ w347]
            tunnel: w328 -> [w340 w344]
            tunnel: [w339 w345] -> w327
            tunnel: [w336 w343] -> w326
            tunnel: w325 -> [w336 w342]
            frame "Constant" {
              n60 = call "IMAQ Xor"("Constant"=w335, "Xor/Xnor (Xor)"=TRUE ("And/Nand (And)"), "error in (no error)"=w340, "Image Dst"=w337, "Image Src A"=w337) -> ("error out"=w339:errorcluster, "Image Dst Out"=w338:T3)  [unwired: 5 in]
            }
            frame "Image", Default {
              n61 = call "IMAQ ReadFile"("File Path"=w347, "error in (no error)"=w344, "Image"=w342) -> ("error out"=w346:errorcluster, "Image Out"=w343:T3)  [unwired: 4 in, 3 out]
              n62 = call "IMAQ Xor"("Xor/Xnor (Xor)"=TRUE ("And/Nand (And)"), "error in (no error)"=w346, "Image Src B"=w343, "Image Dst"=w349, "Image Src A"=w349) -> ("error out"=w345:errorcluster, "Image Dst Out"=w348:T3)  [unwired: 5 in]
            }
          }
        }
        frame "Not Exclusive Or" {
          n63 = case shown="\"Constant\"" w354 {
            tunnel: w358 -> [w360 _]
            tunnel: w357 -> [w362 w374]
            tunnel: [w363 w373] -> w356
            tunnel: w355 -> [_ w372]
            tunnel: w353 -> [w365 w369]
            tunnel: [w364 w370] -> w352
            tunnel: [w361 w368] -> w351
            tunnel: w350 -> [w361 w367]
            frame "Constant" {
              n64 = call "IMAQ Xor"("Constant"=w360, "Xor/Xnor (Xor)"=FALSE ("And/Nand (And)"), "error in (no error)"=w365, "Image Dst"=w362, "Image Src A"=w362) -> ("error out"=w364:errorcluster, "Image Dst Out"=w363:T3)  [unwired: 5 in]
            }
            frame "Image", Default {
              n65 = call "IMAQ ReadFile"("File Path"=w372, "error in (no error)"=w369, "Image"=w367) -> ("error out"=w371:errorcluster, "Image Out"=w368:T3)  [unwired: 4 in, 3 out]
              n66 = call "IMAQ Xor"("Xor/Xnor (Xor)"=FALSE ("And/Nand (And)"), "error in (no error)"=w371, "Image Src B"=w368, "Image Dst"=w374, "Image Src A"=w374) -> ("error out"=w370:errorcluster, "Image Dst Out"=w373:T3)  [unwired: 5 in]
            }
          }
        }
        frame "Logical Difference" {
          n67 = case shown="\"Image\", Default" w379 {
            tunnel: w383 -> [w384 _]
            tunnel: w382 -> [w386 w397]
            tunnel: [w387 w396] -> w381
            tunnel: w380 -> [_ w395]
            tunnel: w378 -> [w389 w392]
            tunnel: [w388 w393] -> w377
            tunnel: [w385 w391] -> w376
            tunnel: w375 -> [w385 w390]
            frame "Constant" {
              n68 = call "IMAQ LogDiff"("Image Src A"=w386, "Constant"=w384, "Image Dst"=w386, "error in (no error)"=w389) -> ("Image Dst Out"=w387:T3, "error out"=w388:errorcluster)  [unwired: 3 in]
            }
            frame "Image", Default {
              n69 = call "IMAQ ReadFile"("File Path"=w395, "error in (no error)"=w392, "Image"=w390) -> ("error out"=w394:errorcluster, "Image Out"=w391:T3)  [unwired: 4 in, 3 out]
              n70 = call "IMAQ LogDiff"("Image Src A"=w397, "Image Dst"=w397, "Image Src B"=w391, "error in (no error)"=w394) -> ("Image Dst Out"=w396:T3, "error out"=w393:errorcluster)  [unwired: 3 in]
            }
          }
        }
        frame "Mask" {
          n71 = case shown="\"Image\", Default" w402 {
            tunnel: w406 -> [_ _]
            tunnel: w405 -> [w408 w417]
            tunnel: [w408 w416] -> w404
            tunnel: w403 -> [_ w415]
            tunnel: w401 -> [w407 w412]
            tunnel: [w407 w413] -> w400
            tunnel: [w409 w411] -> w399
            tunnel: w398 -> [w409 w410]
            frame "Constant" {
            }
            frame "Image", Default {
              n72 = call "IMAQ ReadFile"("File Path"=w415, "error in (no error)"=w412, "Image"=w410) -> ("error out"=w414:errorcluster, "Image Out"=w411:T3)  [unwired: 4 in, 3 out]
              n73 = call "IMAQ Mask"("error in (no error)"=w414, "Image Dst"=w417, "Image Mask"=w411, "Image Src"=w417) -> ("error out"=w413:errorcluster, "Image Dst Out"=w416:T3)  [unwired: 1 in]
            }
          }
        }
      }
      n74 = Bundle By Name(cluster=w52, "Process_Type"=w51, "Parameter"=w50) -> (w49:T6)
    }
    frame "GrayMorphology" {
      n75 = Variant To Data(type=T9 {"Operation"=enum."AutoM", "Structuring Element"=[[1, 1, 1], [1, 1, 1], [1, 1, 1]], "Square/Hexa (Square)"=FALSE, "Number of iterations"=1} ("GrayMorphologyParam"), Variant=w420) -> (data=w433:T9)  [unwired: 1 in, 1 out]
      n76 = Unbundle By Name(w433) -> ("Operation"=w432:T17, "Structuring Element"=w431:i32[][], "Square/Hexa (Square)"=w430:bool, "Number of iterations"=w429:i32)
      n77 = call "IMAQ GrayMorphology"("Number of iterations (1)"=w429, "Structuring Element"=w431, "Square/Hexa (Square)"=w430, "error in (no error)"=w428, "Operation"=w432, "Image Dst"=w426, "Image Src"=w426) -> ("error out"=w427:errorcluster, "Image Dst Out"=w425:T3)  [unwired: 3 in]
      n78 = Bundle By Name(cluster=w424, "Process_Type"=w423, "Parameter"=w420) -> (w422:T6)
    }
    frame "Filters" {
      n79 = Variant To Data(type="FiltersParam", Variant=w435) -> (data=w436:T4)  [unwired: 1 in, 1 out]
      n80 = Unbundle By Name(w436) -> ("FilterFunction"=w454:T18, "Divider"=w445:sgl, "Kernel Size"=w437:i32, "Filter Size X"=w453:i32, "Filter Size Y"=w452:i32, "Tolerance %"=w451:i32, "Kernel"=w446:sgl[][], "Sigma"=w442:sgl, "LThres"=w441:sgl, "HThresh"=w440:sgl, "Windows Size"=w443:i32)
      n81 = case shown="\"Edge Detection - Laplacian\"" w454 {
        tunnel: w453 -> [w465 _ _ w501 _ _ _ _ _ _ _ _ _ _ _ _]
        tunnel: w452 -> [w464 _ _ w500 _ _ _ _ _ _ _ _ _ _ _ _]
        tunnel: w451 -> [w474 _ _ _ _ _ _ _ _ _ _ _ _ _ _ _]
        tunnel: w450 -> [w462 w487 w491 w498 _ w524 w531 w536 w541 w546 w556 w562 w566 _ w574 w578]
        tunnel: [w459 w485 w489 w495 _ w526 w530 w535 w539 w545 w555 w560 w565 _ w573 w577] -> w449
        tunnel: w448 -> [w463 w488 w494 w499 w522 w528 w532 w537 w542 w547 w554 w561 w567 w569 w575 w581]
        tunnel: [w472 w486 w490 w496 w522 w527 w529 w534 w540 w544 w553 w559 w564 w569 w572 w576] -> w447
        tunnel: w446 -> [_ w483 w492 _ _ w523 _ _ _ _ _ _ _ _ w571 w580]
        tunnel: w445 -> [_ w484 w493 _ _ w525 _ _ _ _ _ _ _ _ w570 w579]
        tunnel: w443 -> [_ _ _ _ _ _ _ _ _ _ w552 _ _ _ _ _]
        tunnel: w442 -> [_ _ _ _ _ _ _ _ _ _ w551 _ _ _ _ _]
        tunnel: w441 -> [_ _ _ _ _ _ _ _ _ _ w550 _ _ _ _ _]
        tunnel: w440 -> [_ _ _ _ _ _ _ _ _ _ w549 _ _ _ _ _]
        tunnel: w437 -> [_ _ _ _ _ _ _ _ _ _ _ _ _ _ _ _]
        tunnel: w436 -> [_ _ _ _ _ _ _ _ _ _ _ _ _ _ _ _]
        frame "Smoothing - Low Pass" {
          n82 = Max & Min(x=w465, y=w464) -> (max(x,y)=w466:i32)  [unwired: 1 out]
          n83 = call "IMAQ ImageBorderSize"("Get/Set Status? (Set)"=FALSE, "Image"=w463, "error in (no error)"=w462) -> ("Image Out"=w468:T3, "error out"=w469:errorcluster, "Image border size out"=w470:i32)  [unwired: 1 in]
          n84 = Greater?(x=w466, y=w470) -> (0:w467:bool)
          n85 = case shown="True" w467 {
            tunnel: w469 -> [w475 w481]
            tunnel: w468 -> [w476 w480]
            tunnel: [w476 w479] -> w461
            tunnel: [w475 w478] -> w460
            tunnel: w466 -> [_ w477]
            frame False {
            }
            frame True {
              n86 = call "IMAQ ImageBorderSize"("Get/Set Status? (Set)"=TRUE, "Image"=w480, "Image border size in"=w477, "error in (no error)"=w481) -> ("Image Out"=w479:T3, "error out"=w478:errorcluster)  [unwired: 1 out]
            }
          }
          n87 = Bundle("Filter Size X"=w465, "Filter Size Y"=w464, "Tolerance %"=w474) -> (w473:T19)  [unwired: 1 in]
          n88 = call "IMAQ LowPass"("Image Src"=w461, "Size & Tolerance"=w473, "Image Dst"=w461, "error in (no error)"=w460) -> ("Image Dst Out"=w472:T3, "error out"=w459:errorcluster)  [unwired: 3 in]
        }
        frame "Smoothing - Local Average" {
          n89 = call "IMAQ Convolute"("Kernel"=w483, "Divider (kernel sum)"=w484, "error in (no error)"=w487, "Image Dst"=w488, "Image Src"=w488) -> ("error out"=w485:errorcluster, "Image Dst Out"=w486:T3)  [unwired: 2 in, 3 out]
        }
        frame "Smoothing - Guassian" {
          n90 = call "IMAQ Convolute"("Kernel"=w492, "Divider (kernel sum)"=w493, "error in (no error)"=w491, "Image Dst"=w494, "Image Src"=w494) -> ("error out"=w489:errorcluster, "Image Dst Out"=w490:T3)  [unwired: 2 in, 3 out]
        }
        frame "Smoothing - Median" {
          n91 = call "IMAQ ImageBorderSize"("Get/Set Status? (Set)"=FALSE, "Image"=w499, "error in (no error)"=w498) -> ("Image Out"=w505:T3, "error out"=w506:errorcluster, "Image border size out"=w507:i32)  [unwired: 1 in]
          n92 = Max & Min(x=w501, y=w500) -> (max(x,y)=w502:i32)  [unwired: 1 out]
          n93 = Greater?(x=w502, y=w507) -> (0:w503:bool)
          n94 = case shown="True" w503 {
            tunnel: w506 -> [w514 w520]
            tunnel: w505 -> [w515 w519]
            tunnel: [w515 w518] -> w497
            tunnel: [w514 w517] -> w504
            tunnel: w502 -> [_ w516]
            frame False {
            }
            frame True {
              n95 = call "IMAQ ImageBorderSize"("Get/Set Status? (Set)"=TRUE, "Image"=w519, "Image border size in"=w516, "error in (no error)"=w520) -> ("Image Out"=w518:T3, "error out"=w517:errorcluster)  [unwired: 1 out]
            }
          }
          n96 = Multiply(x=w501, y=w500) -> (x*y=w513:i32)
          n97 = Divide(x=w513, y=2) -> (x/y=w511:dbl)
          n98 = Round Toward -Infinity(1:w511) -> (0:w510:dbl)
          n99 = Bundle("Filter Size X"=w501, "Filter Size Y"=w500, w510) -> (w509:T20)  [unwired: 1 out]
          n100 = call "IMAQ NthOrder"("Image Src"=w497, "Size & Order #"=w509, "Image Dst"=w497, "error in (no error)"=w504) -> ("Image Dst Out"=w496:T3, "error out"=w495:errorcluster)  [unwired: 1 in, 2 out]
        }
        frame "------------------------------------", Default {
        }
        frame "Edge Detection - Laplacian" {
          n101 = call "IMAQ Convolute"("Kernel"=w523, "Divider (kernel sum)"=w525, "error in (no error)"=w524, "Image Dst"=w528, "Image Src"=w528) -> ("error out"=w526:errorcluster, "Image Dst Out"=w527:T3)  [unwired: 2 in, 3 out]
        }
        frame "Edge Detection - Diff" {
          n102 = call "IMAQ EdgeDetection"("Method"=T10."Differentiation", "error in (no error)"=w531, "Image Dst"=w532, "Image Src"=w532) -> ("error out"=w530:errorcluster, "Image Dst Out"=w529:T3)  [unwired: 2 in, 4 out]
        }
        frame "Edge Detection - Prewitt" {
          n103 = call "IMAQ EdgeDetection"("Method"=T10."Prewitt", "error in (no error)"=w536, "Image Dst"=w537, "Image Src"=w537) -> ("error out"=w535:errorcluster, "Image Dst Out"=w534:T3)  [unwired: 2 in, 4 out]
        }
        frame "Edge Detection - Sobel" {
          n104 = call "IMAQ EdgeDetection"("Method"=T10."Sobel", "error in (no error)"=w541, "Image Dst"=w542, "Image Src"=w542) -> ("error out"=w539:errorcluster, "Image Dst Out"=w540:T3)  [unwired: 2 in, 4 out]
        }
        frame "Edge Detection - Roberts" {
          n105 = call "IMAQ EdgeDetection"("Method"=T10."Roberts" ("Method (Filters 1)"), "error in (no error)"=w546, "Image Dst"=w547, "Image Src"=w547) -> ("error out"=w545:errorcluster, "Image Dst Out"=w544:T3)  [unwired: 2 in, 4 out]
        }
        frame "Edge Detection - Canny" {
          w558 = T21 {"Sigma"=1.0, "HThresh"=0.7, "LThres"=0.2, "WindowSize"=9}  # Filter Parameters
          n106 = Bundle By Name(cluster=w558, "Sigma"=w551, "HThresh"=w550, "LThres"=w549, "WindowSize"=w552) -> (w557:T21)
          n107 = call "IMAQ CannyEdgeDetection"("Image Src"=w554, "Image Dst"=w554, "Filter Parameters"=w557, "error in (no error)"=w556) -> ("Image Dst Out"=w553:T3, "error out"=w555:errorcluster)  [unwired: 4 out]
        }
        frame "Edge Detection - Gradient" {
          n108 = call "IMAQ EdgeDetection"("Method"=T10."Gradient" ("Method (Filters 1)"), "error in (no error)"=w562, "Image Dst"=w561, "Image Src"=w561) -> ("error out"=w560:errorcluster, "Image Dst Out"=w559:T3)  [unwired: 2 in, 4 out]
        }
        frame "Edge Detection - Sigma" {
          n109 = call "IMAQ EdgeDetection"("Method"=T10."Sigma" ("Method (Filters 1)"), "error in (no error)"=w566, "Image Dst"=w567, "Image Src"=w567) -> ("error out"=w565:errorcluster, "Image Dst Out"=w564:T3)  [unwired: 2 in, 4 out]
        }
        frame "----------------------------------------" {
        }
        frame "Convolution - Highlight Details" {
          n110 = call "IMAQ Convolute"("Kernel"=w571, "Divider (kernel sum)"=w570, "error in (no error)"=w574, "Image Dst"=w575, "Image Src"=w575) -> ("error out"=w573:errorcluster, "Image Dst Out"=w572:T3)  [unwired: 2 in, 3 out]
        }
        frame "Convolution - Custom" {
          n111 = call "IMAQ Convolute"("Kernel"=w580, "Divider (kernel sum)"=w579, "error in (no error)"=w578, "Image Dst"=w581, "Image Src"=w581) -> ("error out"=w577:errorcluster, "Image Dst Out"=w576:T3)  [unwired: 2 in, 3 out]
        }
      }
      n112 = Bundle By Name(cluster=w457, "Process_Type"=w456, "Parameter"=w435) -> (w455:T6)
    }
    frame "Lookup Table" {
      n113 = Variant To Data(error in=w596, type=T11 {"Function"=enum."Equalizer", "Power Value"=0.0} ("LookupTableParam"), Variant=w585) -> (data=w594:T11, error out=w591:errorcluster)
      n114 = Unbundle By Name(w594) -> ("Function"=w593:T22, "Power Value"=w588:sgl)
      n115 = case shown="\"Reverse\"" w593 {
        tunnel: w592 -> [w601 w612 w618 w622 w628 w634 w640 w647]
        tunnel: w591 -> [w600 w611 w617 w621 w627 w633 w639 w645]
        tunnel: [w599 w610 w615 w619 w625 w631 w638 w644] -> w590
        tunnel: [w598 w609 w616 w620 w626 w632 w637 w643] -> w589
        tunnel: w588 -> [_ _ _ _ _ _ w641 w646]
        frame "Equalizer", Default {
          n116 = call "IMAQ Histogram"("error in (no error)"=w600, "Image"=w601) -> ("error out"=w604:errorcluster, "Histogram Report"=w606:T23)  [unwired: 3 in, 5 out]
          n117 = call "IMAQ GetImageInfo"("error in (no error)"=w604, "Image"=w601) -> ("error out"=w603:errorcluster, "Image Type"=w605:T24)  [unwired: 8 out]
          n118 = case shown="0" w605 {
            tunnel: [cluster{"Minimum":sgl, "Maximum":sgl} {"Minimum"=0.0, "Maximum"=255.0} ("Range") cluster{"Minimum":sgl, "Maximum":sgl} {"Minimum"=0.0, "Maximum"=0.0} ("Range")] -> w602
            frame 0 {
            }
            frame Default {
            }
          }
          n119 = call "IMAQ Equalize"("Range"=w602, "Histogram Report"=w606, "error in (no error)"=w603, "Image Dst"=w601, "Image Src"=w601) -> ("error out"=w599:errorcluster, "Image Dst Out"=w598:T3)  [unwired: 1 in, 4 out]
        }
        frame "Logarithmic" {
          n120 = call "IMAQ MathLookup"("Operator"=T12."Log" ("Operator (Lookup Table 1)"), "X Value"=sgl 1.5 ("X Value (Lookup Table 1)"), "error in (no error)"=w611, "Image Dst"=w612, "Image Src"=w612) -> ("error out"=w610:errorcluster, "Image Dst Out"=w609:T3)  [unwired: 2 in, 3 out]
        }
        frame "Reverse" {
          n121 = call "IMAQ Inverse"("error in (no error)"=w617, "Image Dst"=w618, "Image Src"=w618) -> ("error out"=w615:errorcluster, "Image Dst Out"=w616:T3)  [unwired: 1 in, 6 out]
        }
        frame "Exponential" {
          n122 = call "IMAQ MathLookup"("Operator"=T12."Exp" ("Operator (Lookup Table 1)"), "X Value"=sgl 1.5 ("X Value (Lookup Table 1)"), "error in (no error)"=w621, "Image Dst"=w622, "Image Src"=w622) -> ("error out"=w619:errorcluster, "Image Dst Out"=w620:T3)  [unwired: 2 in, 3 out]
        }
        frame "Square" {
          n123 = call "IMAQ MathLookup"("Operator"=T12."Square" ("Operator (Lookup Table 1)"), "X Value"=sgl 1.5 ("X Value (Lookup Table 1)"), "error in (no error)"=w627, "Image Dst"=w628, "Image Src"=w628) -> ("error out"=w625:errorcluster, "Image Dst Out"=w626:T3)  [unwired: 2 in, 3 out]
        }
        frame "Square Root" {
          n124 = call "IMAQ MathLookup"("Operator"=T12."Square root" ("Operator (Lookup Table 1)"), "X Value"=sgl 1.5 ("X Value (Lookup Table 1)"), "error in (no error)"=w633, "Image Dst"=w634, "Image Src"=w634) -> ("error out"=w631:errorcluster, "Image Dst Out"=w632:T3)  [unwired: 2 in, 3 out]
        }
        frame "Power X" {
          n125 = call "IMAQ MathLookup"("Operator"=T12."Power X" ("Operator (Lookup Table 1)"), "X Value"=w641, "error in (no error)"=w639, "Image Dst"=w640, "Image Src"=w640) -> ("error out"=w638:errorcluster, "Image Dst Out"=w637:T3)  [unwired: 2 in, 3 out]
        }
        frame "Power 1/X" {
          n126 = call "IMAQ MathLookup"("Operator"=T12."Power 1/X" ("Operator (Lookup Table 1)"), "X Value"=w646, "error in (no error)"=w645, "Image Dst"=w647, "Image Src"=w647) -> ("error out"=w644:errorcluster, "Image Dst Out"=w643:T3)  [unwired: 2 in, 3 out]
        }
      }
      n127 = Bundle By Name(cluster=w587, "Process_Type"=w584, "Parameter"=w585) -> (w586:T6)
    }
    frame "Particle Filter" {
      n128 = Variant To Data(error in=w666, type=T13 {"Selection Values"=[{"Measurement Parameter"=0, "Range Lower Value"=0.0, "Range Upper Value"=0.0, "Range"=FALSE, "Measurement Type"=FALSE}], "Keep/Remove Particles (F)"=FALSE, "Reject Border? (F)"=FALSE, "Fill Holes? (F)"=FALSE, "Connectivity 4/8 (8)"=FALSE} ("ParticleFilterParam"), Variant=w662) -> (data=w665:T13, error out=w659:errorcluster)
      n129 = Unbundle By Name(w665) -> ("Selection Values"=w656:T25, "Keep/Remove Particles (F)"=w651:bool, "Reject Border? (F)"=w653:bool, "Fill Holes? (F)"=w652:bool, "Connectivity 4/8 (8)"=w655:bool)
      n130 = call "IMAQ Particle Filter 3"("Image Src"=w657, "Connectivity 4/8 (8)"=w655, "Image Dst"=w657, "Selection Values"=w656, "Keep/Remove Particles (F)"=w651, "error in (no error)"=w659, "Reject Border? (F)"=w653, "Fill Holes? (F)"=w652) -> ("Image Dst Out"=w658:T3, "error out"=w654:errorcluster)  [unwired: 5 in, 1 out]
      n131 = Bundle By Name(cluster=w664, "Process_Type"=w661, "Parameter"=w662) -> (w663:T6)
    }
    frame "None", Default {
    }
    frame "Mask" {
      w678 = T26 {"Function"=enum."Inside", "ROI List"=0, "ROI"=[], "Creat ROI"=FALSE, "Delete ROI"=FALSE, "Enabled/Disabled"=FALSE, "Color Box"=0, "Last Mouse Position"={"X"=0, "Y"=0}}  # MaskParam
      w683 = T24 0 items=["Grayscale (U8)", "Grayscale (I16)", "Grayscale (SGL)", "Complex (CSG)", "RGB (U32)", "HSL (U32)", "RGB (U64)", "Grayscale (U16)"] ("y")
      n132 = call "IMAQ GetImageInfo"("Image"=w673) -> ("Image Type"=w684:T24)  [unwired: 3 in, 7 out]
      n133 = Not Equal?(x=w684, y=w683) -> (x != y?=w676:bool)
      n134 = case shown="False" w676 {
        tunnel: w679 -> [w704 _]
        tunnel: [w697 w796] -> w687
        tunnel: w686 -> [w689 _]
        tunnel: [w702 errorcluster {"status"=TRUE, "code"=0, "source"=""} ("error out")] -> w685
        tunnel: w673 -> [w701 w796]
        tunnel: w678 -> [w698 _]
        tunnel: w673 -> [w696 _]
        tunnel: w675 -> [w694 w795]
        tunnel: [w690 w795] -> w674
        frame False {
          n135 = Variant To Data(type=w698, Variant=w704) -> (data=w703:T26)  [unwired: 1 in, 1 out]
          n136 = Unbundle By Name(w703) -> ("Function"=w695:enum16{"Inside", "Outside"}, "ROI"=w699:T27, "Last Mouse Position"=w693:cluster{"X":i32, "Y":i32}, "Color Box"=w691:u32, "Enabled/Disabled"=w692:bool)
          n137 = Empty Array?(array=w699) -> (empty?=w700:bool)
          n138 = case shown="False" w700 {
            tunnel: w689 -> [w716 w781]
            tunnel: [_ w781] -> w702
            tunnel: w701 -> [w708 w794]
            tunnel: w699 -> [w717 _]
            tunnel: [w706 w794] -> w697
            tunnel: w696 -> [w707 w788]
            tunnel: w695 -> [w715 _]
            tunnel: w694 -> [w714 w787]
            tunnel: w693 -> [w713 w786]
            tunnel: w692 -> [w705 _]
            tunnel: w691 -> [w711 _]
            tunnel: [w712 w782] -> w690
            tunnel: w689 -> [_ _]
            frame False {
              n139 = for {
                tunnel: w717 -> [w755] mode=indexing
                tunnel: w716 -> [w757]
                tunnel: w708 -> [w756]
                tunnel: w707 -> [w742]
                shift-right: [w747] -> w709
                shift-left: i32[][] [] -> [w750]
                tunnel: w715 -> [w746]
                tunnel: w705 -> [w741]
                tunnel: w711 -> [w739]
                i -> [w752]
                w760 = T24 0 items=["Grayscale (U8)", "Grayscale (I16)", "Grayscale (SGL)", "Complex (CSG)", "RGB (U32)", "HSL (U32)", "RGB (U64)", "Grayscale (U16)"] ("Image Type")
                n140 = Number To Decimal String(number=w752) -> (decimal integer string=w761:string)  [unwired: 1 in]
                n141 = Equal To 0?(x=w752) -> (x = 0?=w751:bool)
                n142 = Concatenate Strings("Mask Image", w761) -> (w759:string)
                n143 = call "IMAQ Create"("Image Name"=w759, "Image Type"=w760, "error in (no error)"=w757) -> ("New Image"=w758:T3, "error out"=w734:errorcluster)  [unwired: 2 in]
                n144 = Select(t=w739, s=w741, f=u8 0) -> (s? t:f=w738:u32)
                n145 = call "IMAQ ROIToMask 2"("Background Value (0)"=w738, "Image Model"=w756, "error in (no error)"=w734, "ROI Descriptor"=w755, "Image"=w758) -> ("error out"=w735:errorcluster, "Image Out"=w754:T3)  [unwired: 4 in, 1 out]
                n146 = call "IMAQ ImageToArray"("error in (no error)"=w735, "Image"=w754) -> ("error out"=w733:errorcluster, "Image Pixels (U8)"=w737:u8[][])  [unwired: 2 in, 3 out]
                n147 = call "Replace Mask Element.vi"("Numeric"=i16 255, "Array"=w737, "error in (no error)"=w733) -> ("row"=w749:i32, "col"=w748:i32, "error out"=w732:errorcluster)  [unwired: 9 in, 1 out]
                n148 = call-poly "IMAQ Extract Tetragon"("error in (no error)"=w732, "ROI Descriptor"=w755, "Image Dst"=w754, "Image Src"=w742) -> ("error out"=w731:errorcluster, "Image Dst Out"=w753:T3)  [unwired: 6 in]
                n149 = call "IMAQ ImageToArray"("error in (no error)"=w731, "Image"=w753) -> ("Image Pixels (U8)"=w744:u8[][])  [unwired: 2 in, 4 out]
                n150 = case shown="\"Outside\"" w746 {
                  tunnel: w737 -> [w764 w765]
                  tunnel: [w764 w769] -> w745
                  tunnel: w744 -> [w763 w768]
                  tunnel: [w763 w766] -> w743
                  tunnel: w742 -> [_ w770]
                  frame "Inside", Default {
                  }
                  frame "Outside" {
                    w767 = 0 ("index (row)")
                    n151 = call "IMAQ ImageToArray"("Image"=w770) -> ("Image Pixels (U8)"=w769:u8[][])  [unwired: 3 in, 4 out]
                    n152 = Replace Array Subset(array=w768, new element=w765, index (row)=w767, index (col)=w767) -> (w766:u8[][])
                  }
                }
                n153 = case shown="False" w751 {
                  tunnel: w750 -> [w775 _]
                  tunnel: w745 -> [_ w780]
                  tunnel: w749 -> [w774 w779]
                  tunnel: w748 -> [w773 w778]
                  tunnel: w743 -> [w772 w777]
                  tunnel: [w771 w776] -> w747
                  frame False {
                    n154 = Replace Array Subset(array=w775, new element=w772, index (row)=w774, index (col)=w773) -> (w771:i32[][])
                  }
                  frame True {
                    n155 = Replace Array Subset(array=w780, new element=w777, index (row)=w779, index (col)=w778) -> (w776:u8[][])
                  }
                }
              }
              n156 = call "IMAQ ArrayToImage"("Image Pixels (U8)"=w709, "Image"=w708) -> ("Image Out"=w706:T3)  [unwired: 8 in, 1 out]
              n157 = case shown="False" w705 {
                tunnel: w714 -> [w729 w730]
                tunnel: w713 -> [w726 _]
                tunnel: [w719 w730] -> w712
                tunnel: w706 -> [w718 _]
                frame False {
                  w721 = refnum<vi> refnum  # ColorBox
                  n158 = Unbundle By Name(w726) -> ("X"=w725:i32, "Y"=w724:i32)
                  n159 = property class="Clust (strict)"(reference=w729) -> (reference out=w719:refnum<vi>, "Controls[]"=w728:refnum<vi>[])  [unwired: 1 in, 1 out]
                  n160 = call "IMAQ GetPixelValue"("Image"=w718, "X Coordinate"=w725, "Y Coordinate"=w724) -> ("Pixel Value (U8)"=w723:u8)  [unwired: 3 in, 4 out]
                  n161 = Index Array(array=w728, index=6) -> (element=w722:refnum<vi>)
                  n162 = To More Specific Class(target class=w721, reference=w722) -> (specific class reference=w720:refnum<vi>)  [unwired: 1 in, 1 out]
                  n163 = property class="ColBox"(reference=w720, "Value"=w723) -> ()  [unwired: 1 in, 2 out]
                }
                frame True {
                }
              }
            }
            frame True {
              w784 = refnum<vi> refnum  # ColorBox
              n164 = Unbundle By Name(w786) -> ("X"=w791:i32, "Y"=w790:i32)
              n165 = property class="Clust (strict)"(reference=w787) -> (reference out=w782:refnum<vi>, "Controls[]"=w793:refnum<vi>[])  [unwired: 1 in, 1 out]
              n166 = call "IMAQ GetPixelValue"("Image"=w788, "X Coordinate"=w791, "Y Coordinate"=w790) -> ("Pixel Value (U8)"=w789:u8)  [unwired: 3 in, 4 out]
              n167 = Index Array(array=w793, index=6) -> (element=w785:refnum<vi>)
              n168 = To More Specific Class(target class=w784, reference=w785) -> (specific class reference=w783:refnum<vi>)  [unwired: 1 in, 1 out]
              n169 = property class="ColBox"(reference=w783, "Value"=w789) -> ()  [unwired: 1 in, 2 out]
            }
          }
        }
        frame True {
        }
      }
      n170 = Bundle By Name(cluster=w682, "Process_Type"=w680, "Parameter"=w679) -> (w681:T6)
    }
  }
  "error out" <- w11
  "Image Out" <- w10
  "ProcessSettingOut" <- w9
  "OperatorImageOut" <- w5
  "ExtractImage" <- w4
  "MaskParam 4" <- w1
